vi "Initialize.vi"(8 "error in (no error)":errorcluster, 10 "Physical Camera Assignment":T1[](array[typedef])) -> (0 "error out":errorcluster, 3 "Orca-Flash 4.0 out":refnum<class "Hamamatsu Camera.lvclass">)   [LabVIEW 2018, in "Hamamatsu Camera.lvlib" / "Hamamatsu Camera.lvclass"]
uses:
  Hamamatsu Camera.lvclass
  C:/FlashGordon/Development/Hardware/Camera/Camera.lvclass
  Resources/Type Defs/Physical Camera Assignment.ctl
  Resources/Type Defs/Camera Type.ctl
  Hamamatsu Camera.lvclass/Hamamatsu Camera.ctl
  Resources/GLOBAL/GLOBAL Time-critical.vi
panel:
  out "Camera Details Array":T3(array[cluster])
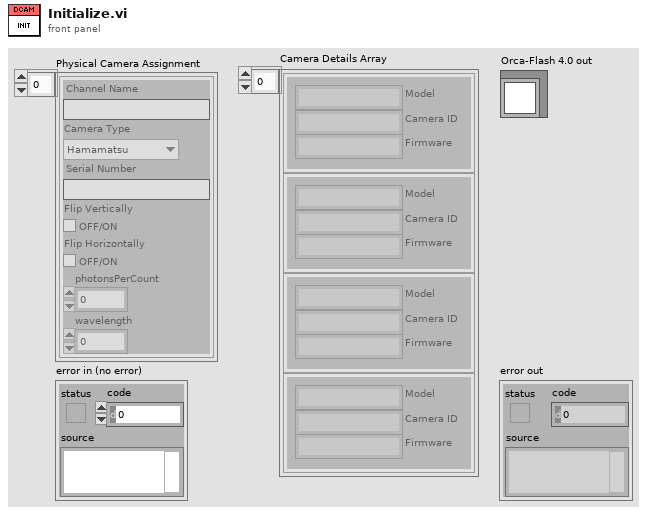
[diagram p1: front panel]
types:
  T1 = typedef "Physical Camera Assignment.ctl" = cluster{"Channel Name":string, "Camera Type":T2, "Serial Number":string, "Flip Vertically":bool, "Flip Horizontally":bool, "photonsPerCount":dbl, "wavelength":i16}
  T2 = typedef "Camera Type.ctl" = enum16{"Hamamatsu"}
  T3 = cluster{"Model":string, "Camera ID":string, "Firmware":string}[]
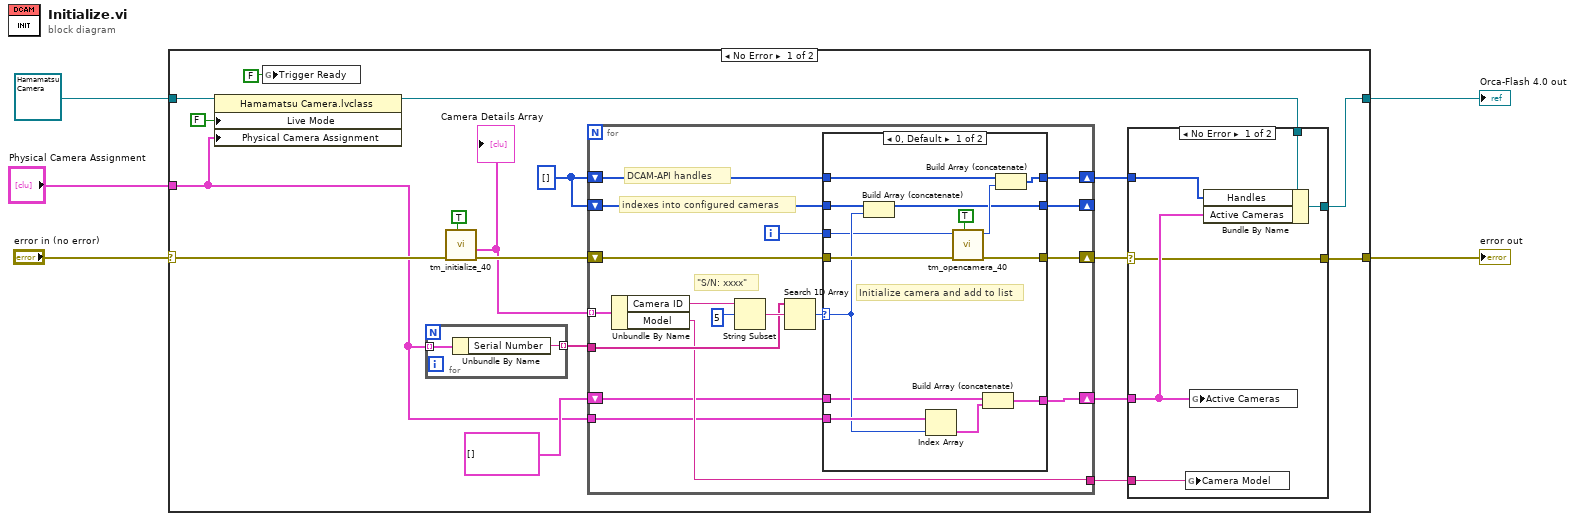
[diagram p0: block diagram]
diagram:
  n1 = case shown="No Error" "error in (no error)" {
    selector: "error in (no error)" -> [w23 w70]
    tunnel: [w7 w70] -> w3
    tunnel: refnum<class "Hamamatsu Camera.lvclass"> refnum ("Hamamatsu Camera.lvlib:Hamamatsu Camera.lvclass") -> [w16 w69]
    tunnel: [w22 w69] -> w4
    tunnel: "Physical Camera Assignment" -> [w6 _]
    frame No Error {
      w19 = u32[] []
      n2 = property class="Hamamatsu Camera.lvclass"(reference=w16, "Live Mode"=FALSE, "Physical Camera Assignment"=w6) -> (reference out=w15:refnum<class "Hamamatsu Camera.lvclass">)  [unwired: 1 in, 1 out]
      n3 = global write "GLOBAL Time-critical.vi" "Trigger Ready"(FALSE) -> ()
      n4 = for {
        tunnel: w6 -> [w68] mode=indexing
        tunnel: [w67] -> w21 mode=indexing
        n5 = Unbundle By Name(w68) -> ("Serial Number"=w67:string)
      }
      n6 = call <userlib>:"tm_initialize_40.vi"("HVCC Log (F)"=TRUE, "error in (no error)"=w23) -> ("error out"=w20:errorcluster, "Camera Details Array"=w9:T3)  [unwired: 6 in, 2 out]
      "Camera Details Array" <- w9
      n7 = for {
        tunnel: w9 -> [w48] mode=indexing
        tunnel: w21 -> [w44]
        shift-right: [w41] -> w8
        shift-left: w20 -> [w42]
        shift-right: [w40] -> w17
        shift-left: w19 -> [w37]
        shift-right: [w38] -> _
        shift-left: w19 -> [w39]
        tunnel: [w36] -> w18
        tunnel: w6 -> [w34]
        shift-right: [w35] -> w10
        shift-left: T1[] [] -> [w33]
        i -> [w32]
        # "indexes into configured cameras"
        # "DCAM-API handles"
        # "\"S/N: xxxx\""
        n8 = Unbundle By Name(w48) -> ("Camera ID"=w47:string, "Model"=w36:string)
        n9 = String Subset(string=w47, offset (0)=5) -> (substring=w45:string)  [unwired: 1 in]
        n10 = Search 1D Array(1D array=w44, element=w45) -> (index of element=w43:i32)  [unwired: 1 in]
        n11 = case shown="0, Default" w43 {
          selector: w43 -> [w53 _]
          tunnel: w42 -> [w62 w66]
          tunnel: [w61 w66] -> w41
          tunnel: w37 -> [w57 w65]
          tunnel: [w58 w65] -> w40
          tunnel: w39 -> [w55 w64]
          tunnel: [w54 w64] -> w38
          tunnel: [w52 w63] -> w35
          tunnel: w34 -> [w59 _]
          tunnel: w33 -> [w50 w63]
          tunnel: w32 -> [w49 _]
          frame 0, Default {
            # "Initialize camera and add to list"
            n12 = Build Array (concatenate)(w55, w53) -> (w54:u32[])
            n13 = Index Array(array=w59, index=w53) -> (element=w51:T1)
            n14 = call <userlib>:"tm_opencamera_40.vi"("Force Open"=TRUE, "error in (no error)"=w62, "Camera Index"=w49) -> ("error out"=w61:errorcluster, "Handle out"=w56:u32)  [unwired: 6 in, 1 out]
            n15 = Build Array (concatenate)(w50, w51) -> (w52:T1[])
            n16 = Build Array (concatenate)(w57, w56) -> (w58:u32[])
          }
          frame -1 {
            # "camera not found in config file."
          }
        }
      }
      n17 = case shown="No Error" w8 {
        selector: w8 -> [w24 w30]
        tunnel: [w29 w31] -> w22
        tunnel: w18 -> [w28 _]
        tunnel: w17 -> [w27 _]
        tunnel: w15 -> [w26 w31]
        tunnel: w10 -> [w25 _]
        tunnel: [w24 w30] -> w7
        frame No Error {
          n18 = global write "GLOBAL Time-critical.vi" "Camera Model"(w28) -> ()
          n19 = global write "GLOBAL Time-critical.vi" "Active Cameras"(w25) -> ()
          n20 = Bundle By Name(cluster=w26, "Handles"=w27, "Active Cameras"=w25) -> (w29:refnum<class "Hamamatsu Camera.lvclass">)
        }
        frame Error {
          # "Not setting active cameras\nso Application knows that\nstartup has failed."
        }
      }
    }
    frame Error {
    }
  }
  "error out" <- w3
  "Orca-Flash 4.0 out" <- w4
